vi "BME_DG_Gate_AB.vi"(8 "error in (no error)":errorcluster, 10 "Gate AB":bool=TRUE, 11 "DG_Number":i32) -> (0 "error out":errorcluster, 3 "return value":i32)   [LabVIEW 2009, in "POLARIS BME DG.lvlib"]
uses:
  POLARIS BME DG.lvlib
  BME DLL/DelayGenerator.dll
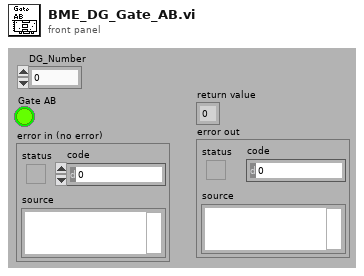
[diagram p1: front panel]
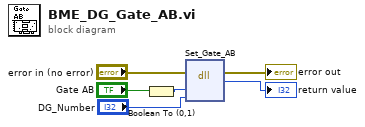
[diagram p0: block diagram]
diagram:
  n1 = Boolean To (0,1)(Boolean="Gate AB") -> (0, 1=w5:i16)
  n2 = dll-call lib="C:/CS Framework/LVSCC/LV2009/GPL/Projects/cs-framework/CSClass/CSPOLARIS/POLARIS BME DG/BME DLL/DelayGenerator.dll" fn="Set_Gate_AB"(error in="error in (no error)", "Gate_AB"=w5, "DG_Number"="DG_Number") -> (error out=→"error out":errorcluster, →"return value":i32)  [unwired: 4 in, 1 out]
